vi "Overlay Custom Arc.vi"(7 "Offset":i32, 9 "Results":T1, 10 "Search Area":enum32{"Upper", "Lower"}(ring), 11 "Refnum in":T2) -> (3 "Refnum out":T2)   [LabVIEW 2015]
uses:
  <vilib>/vision/Image Controls.llb/IMAQ Image.ctl
  controls/Results.ctl
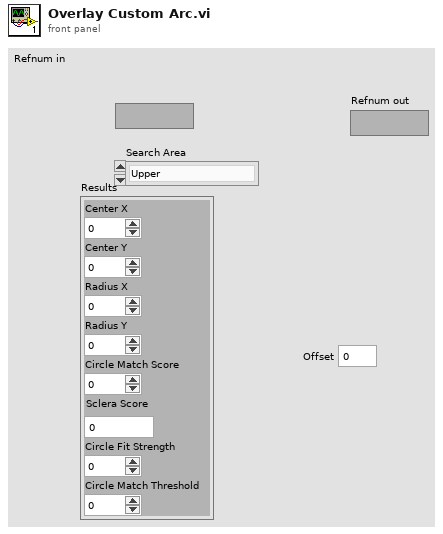
[diagram p1: front panel]
types:
  T1 = typedef "Results.ctl" = cluster{"Center X":i32, "Center Y":i32, "Radius X":i32, "Radius Y":i32, "Circle Match Score":i32, "Sclera Score":dbl, "Circle Fit Strength":i32, "Circle Match Threshold":i32}
  T2 = typedef "IMAQ Image.ctl" = refnum<image>
  T3 = cluster{"Left":i32, "Top":i32, "Right":i32, "Bottom":i32}
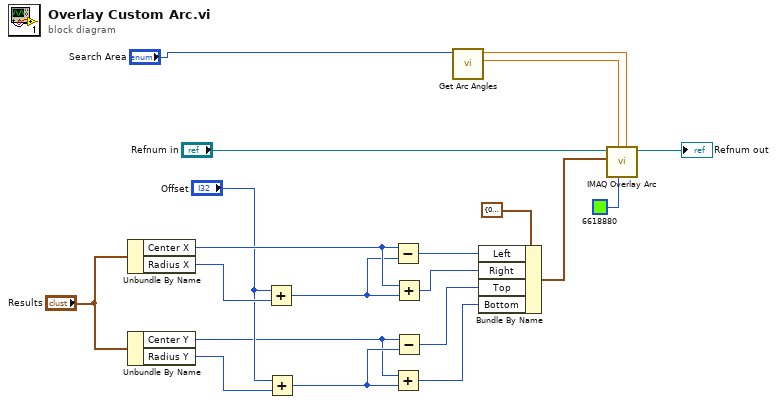
[diagram p0: block diagram]
diagram:
  n1 = Unbundle By Name("Results") -> ("Center X"=w13:i32, "Radius X"=w12:i32)
  n2 = Unbundle By Name("Results") -> ("Center Y"=w2:i32, "Radius Y"=w1:i32)
  n3 = Add(x="Offset", y=w12) -> (x+y=w6:i32)
  n4 = Add(x="Offset", y=w1) -> (x+y=w5:i32)
  n5 = Subtract(x=w13, y=w6) -> (x-y=w11:i32)
  n6 = Add(x=w2, y=w5) -> (x+y=w8:i32)
  n7 = Add(x=w13, y=w6) -> (x+y=w10:i32)
  n8 = Subtract(x=w2, y=w5) -> (x-y=w9:i32)
  n9 = call "Get Arc Angles.vi"("Search Area"="Search Area") -> ("Start Angle (degrees)"=w18:dbl, "End Angle (degrees)"=w19:dbl)  [unwired: 9 in]
  n10 = Bundle By Name(cluster=T3 {"Left"=0, "Top"=0, "Right"=0, "Bottom"=0} ("Bounding Rectangle"), "Left"=w11, "Right"=w10, "Top"=w9, "Bottom"=w8) -> (w7:T3)
  n11 = call "IMAQ Overlay Arc"("End Angle (degrees)"=w19, "Color"=u32 6618880, "Start Angle (degrees)"=w18, "Bounding Rectangle"=w7, "Image"="Refnum in") -> ("Image Out"=→"Refnum out":T2)  [unwired: 5 in, 1 out]
